vi "problem2_part5.vi"() -> ()   [LabVIEW 2020]
panel:
  in  "Height":dbl
  in  "Velocity":dbl
  out "Range of \nProjectile":dbl
  in  "Angle (Radians)":dbl
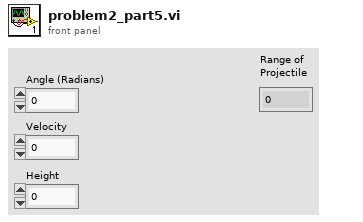
[diagram p1: front panel]
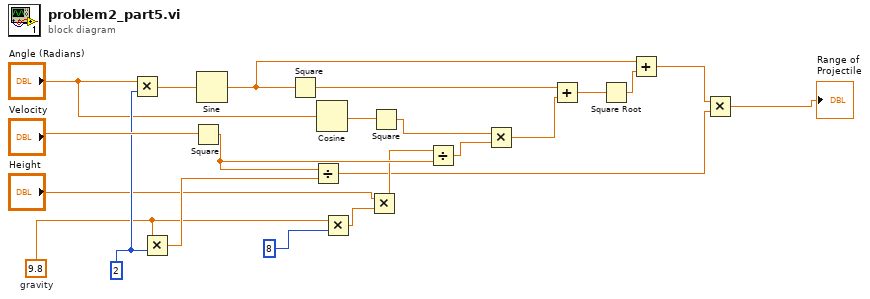
[diagram p0: block diagram]
diagram:
  w20 = 2
  w15 = 9.8  # gravity
  n1 = Multiply(x="Angle (Radians)", y=w20) -> (x*y=w18:dbl)
  n2 = Multiply(x=w15, y=w20) -> (x*y=w21:dbl)
  n3 = Square(x="Velocity") -> (x^2=w11:dbl)
  n4 = Sine(x=w18) -> (sin(x)=w19:dbl)
  n5 = Square(x=w19) -> (x^2=w6:dbl)
  n6 = Divide(x=w11, y=w21) -> (x/y=w2:dbl)
  n7 = Cosine(x="Angle (Radians)") -> (cos(x)=w16:dbl)
  n8 = Multiply(x=w15, y=8) -> (x*y=w12:dbl)
  n9 = Multiply(x="Height", y=w12) -> (x*y=w10:dbl)
  n10 = Square(x=w16) -> (x^2=w8:dbl)
  n11 = Divide(x=w10, y=w11) -> (x/y=w9:dbl)
  n12 = Multiply(x=w8, y=w9) -> (x*y=w7:dbl)
  n13 = Add(x=w6, y=w7) -> (x+y=w5:dbl)
  n14 = Square Root(x=w5) -> (sqrt(x)=w4:dbl)
  n15 = Add(x=w19, y=w4) -> (x+y=w3:dbl)
  n16 = Multiply(x=w3, y=w2) -> (x*y=→"Range of \nProjectile":dbl)
